vi "Test_WriteInteger_NoFormatString_WriteIntegerAsString.vi"(8 "error in (no error)":errorcluster, 11 "TestBooleanTextBinding In":refnum<class "TestBooleanTextBinding.lvclass">) -> (0 "error out":errorcluster, 3 "TestBooleanTextBinding Out":refnum<class "TestBooleanTextBinding.lvclass">)   [LabVIEW 2017, in "TestBooleanTextBinding.lvclass"]
uses:
  TestBooleanTextBinding.lvclass
  Source/Concrete/BooleanTextBinding/BooleanTextBinding.lvclass/BooleanTextBinding.ctl
  Source/Concrete/BooleanTextBinding/BooleanTextBinding.lvclass
  C:/Git/composed-transport/Source/ITransport/ITransport.lvclass
  <vilib>/Utility/error.llb/Error Cluster From Error Code.vi
  Source/ITransport/ITransport.lvclass
panel:
  in  "OK Button":bool
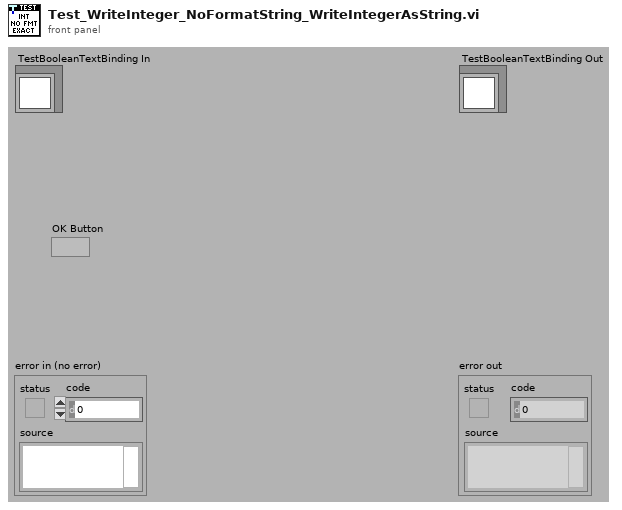
[diagram p1: front panel]
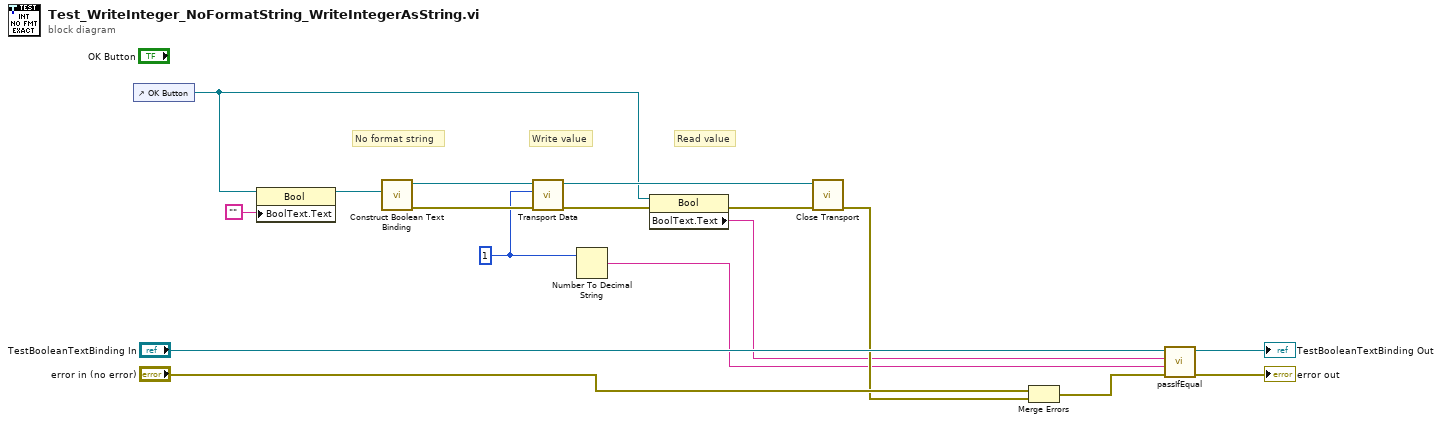
[diagram p0: block diagram]
diagram:
  w2 = 1 ("Format String")
  # "Read value"
  # "No format string"
  # "Write value"
  n1 = control-ref of="OK Button"() -> (w3:refnum<vi>)
  n2 = property class="Bool"(reference=w3, "BoolText.Text"="") -> (reference out=w8:refnum<vi>)  [unwired: 1 in, 1 out]
  n3 = call "Construct Boolean Text Binding.vi"("Bool Refnum"=w8) -> ("error out"=w17:errorcluster, "BooleanTextBinding"=w12:refnum<class "BooleanTextBinding.lvclass">)  [unwired: 9 in]
  n4 = call "Transport Data.vi"("error in (no error)"=w17, "Value"=w2, "ITransport in"=w12) -> ("error out"=w6:errorcluster, "ITransport out"=w10:refnum<class "BooleanTextBinding.lvclass">)  [unwired: 7 in]
  n5 = Number To Decimal String(number=w2) -> (decimal integer string=w1:string)  [unwired: 1 in]
  n6 = property class="Bool"(reference=w3, error in=w6) -> (error out=w5:errorcluster, "BoolText.Text"=w4:string)  [unwired: 1 out]
  n7 = call-dynamic "Close Transport.vi"("error in (no error)"=w5, "ITransport in"=w10) -> ("error out"=w9:errorcluster)  [unwired: 9 in]
  n8 = Merge Errors("error in (no error)", w9) -> (w11:errorcluster)
  n9 = call-dynamic "passIfEqual.vi"("error in (no error)"=w11, "y"=w1, "x"=w4, "TestCase in"="TestBooleanTextBinding In") -> ("error out"=→"error out":errorcluster, "TestCase out"=→"TestBooleanTextBinding Out":refnum<class "TestBooleanTextBinding.lvclass">)  [unwired: 6 in]
